vi "main.vi"() -> ()   [LabVIEW 2022 SP3]
panel:
  out "error out":errorcluster
  in  "String Array":string[](array[string])
  out "Risposta Server":string[](array[string])
  in  "Control":T1(array[cluster])=[{"Device"=10, "Operation"=0, "Command/byte count"="OUTP:LOAD INF\nAPPL:SIN 1000,10,0"}, {"Device"=1, "Operation"=0, "Command/byte count"="HEAD OFF\nDAT:SOU CH1\nDAT:ENC ASCI\nDAT:WID 1\nDAT:STAR 1\nDAT:STOP 2500\nCURV?"}, {"Device"=1, "Operation"=1, "Command/byte count"="15000"}] {"Operation" items=["write", "read"]; "Device" items=["DSO"=1, "AWG"=10]}
  in  "error in (no error)":errorcluster
  in  "Enum":enum16{"55", "56"}(ring)
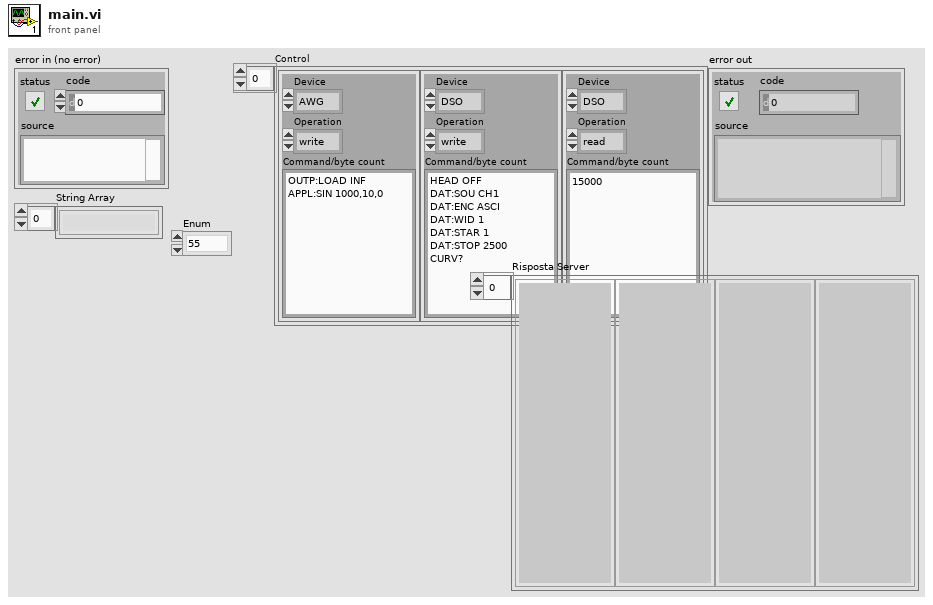
[diagram p1: front panel]
types:
  T1 = cluster{"Device":u16, "Operation":u16, "Command/byte count":string}[]
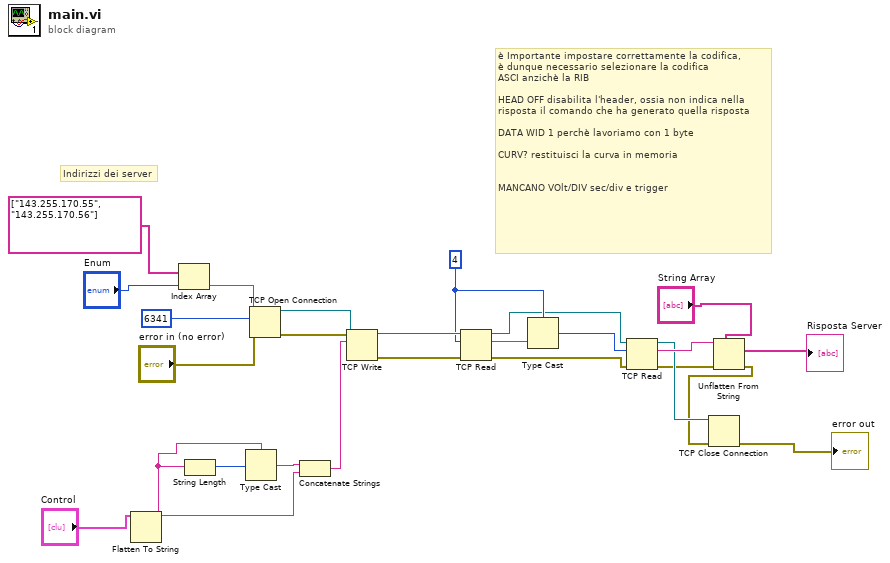
[diagram p0: block diagram]
diagram:
  w13 = 4
  # "è Importante impostare correttamente la codifica,\nè dunque necessario selezionare la codifica \nASCI anzichè la RIB\n\nHEAD OFF disabilita l'header, ossia non indica nella \nrisposta il comando che ha generato quella risposta\n\nDATA WID 1 perchè lavoriamo con 1 byte\n\nCURV? restituisci la curva in memoria\n\n\nMANCANO VOlt/DIV sec/div e trigger"
  # "Indirizzi dei server"
  n1 = Flatten To String(anything="Control") -> (data string=w16:string)  [unwired: 3 in, 2 out]
  n2 = Index Array(array=string[] ["143.255.170.55", "143.255.170.56"], index="Enum") -> (element=w23:string)
  n3 = String Length(string=w16) -> (length=w18:i32)
  n4 = Type Cast(type=w16, x=w18) -> (*(type *) &x=w17:string)
  n5 = TCP Open Connection(address=w23, remote port or service name=u16 6341, error in (no error)="error in (no error)") -> (connection ID=w20:refnum<k5>, error out=w22:errorcluster)  [unwired: 2 in]
  n6 = Concatenate Strings(w17, w16) -> (w5:string)
  n7 = TCP Write(connection ID=w20, data in=w5, error in (no error)=w22) -> (connection ID out=w14:refnum<k5>, error out=w15:errorcluster)  [unwired: 1 in, 1 out]
  n8 = TCP Read(connection ID=w14, bytes to read=w13, error in (no error)=w15) -> (connection ID out=w7:refnum<k5>, data out=w12:string, error out=w10:errorcluster)  [unwired: 2 in]
  n9 = Type Cast(type=w13, x=w12) -> (*(type *) &x=w8:i32)
  n10 = TCP Read(connection ID=w7, bytes to read=w8, error in (no error)=w10) -> (connection ID out=w4:refnum<k5>, data out=w11:string, error out=w2:errorcluster)  [unwired: 2 in]
  n11 = Unflatten From String(type="String Array", binary string=w11, error in (no error)=w2) -> (value=→"Risposta Server":string[], error out=w1:errorcluster)  [unwired: 2 in, 1 out]
  n12 = TCP Close Connection(connection ID=w4, error in (no error)=w1) -> (error out=→"error out":errorcluster)  [unwired: 1 in, 1 out]
